vi "Create.vi"(8 "error in (no error)":errorcluster, 10 "Append Index (-1)":i32=-1, 11 "File Type":T1) -> (0 "error out":errorcluster, 3 "Data out":refnum<class "LV-Data.lvclass">)   [LabVIEW 2019, in "LV-Data.lvclass"]
uses:
  LV-Data.lvclass
  Typedefs/File Type--enum.ctl
  LV-Data.DAT/LV-Data.DAT.lvclass
  C:/Users/patrick/Documents/GitHub/LV-Data/src/LV-Data/LV-Data.lvclass
  LV-Data.ITX/LV-Data.ITX.lvclass
  LV-Data.TDMS/LV-Data.TDMS.lvclass
  LV-Data.lvclass/LV-Data.ctl
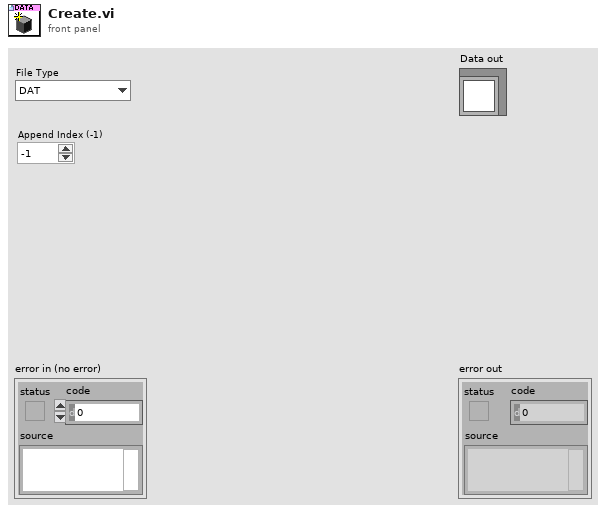
[diagram p1: front panel]
types:
  T1 = typedef "LV-Data.lvclass/File Type--enum.ctl" = enum16{"DAT", "ITX", "TDMS", "VI"}
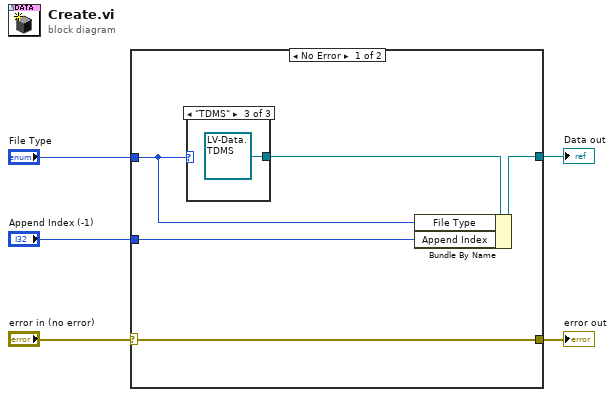
[diagram p0: block diagram]
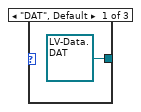
[diagram p2: hidden frame]
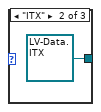
[diagram p3: hidden frame]
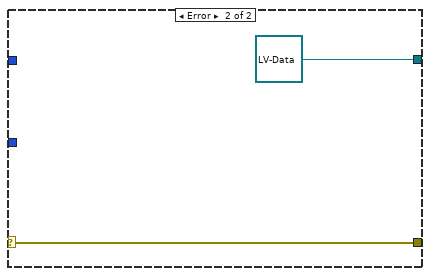
[diagram p4: hidden frame]
diagram:
  n1 = case shown="No Error" "error in (no error)" {
    selector: "error in (no error)" -> [w10 w15]
    tunnel: [w10 w15] -> w4
    tunnel: [w9 refnum<class "LV-Data.lvclass"> refnum ("ITX")] -> w3
    tunnel: "File Type" -> [w7 _]
    tunnel: "Append Index (-1)" -> [w8 _]
    frame No Error {
      n2 = case shown="\"TDMS\"" w7 {
        tunnel: [refnum<class "LV-Data.DAT.lvclass"> refnum ("DAT.lvclass") refnum<class "LV-Data.ITX.lvclass"> refnum ("ITX") refnum<class "LV-Data.TDMS.lvclass"> refnum ("Data.TDMS.lvclass")] -> w6
        frame "DAT", Default {
        }
        frame "ITX" {
        }
        frame "TDMS" {
        }
      }
      n3 = Bundle By Name(cluster=w6, "File Type"=w7, "Append Index"=w8) -> (w9:refnum<class "LV-Data.lvclass">)
    }
    frame Error {
    }
  }
  "error out" <- w4
  "Data out" <- w3
